vi "WS1050 BURN EFUSE Update.vi"() -> ()   [LabVIEW 2009]
panel:
  in  "A364X_VDD":refnum<visa-resource-name>="GPIB1::6::INSTR"
  in  "READBACK":bool
  out "error out 2":errorcluster
  out "Fuse Readback":string
  in  "BIT TO BURN":string="07450F"
  in  "stop":bool
  out "VISA resource name out":refnum<visa-resource-name>
  out "error out":errorcluster
  in  "error in (no error)":errorcluster
  in  "VISA resource name":refnum<visa-resource-name>="COM1"
  in  "PUSH BUTTON \nTO START TEST":bool
  # "TEST PROCEDURE TO BURN FUSE T7\n\n1. BIT TO BURN \"ENTER 0745XX\"\n2. INCREASE VDD TO 5V \"JUMPER THE YELLOW WIRE TO 5V\"\n3. DECREASE VDD TO 3.3V THEN MOVE JUMPER TO GND\n4. COMPLETED\n5. READ BACK TO VERIFY FUSE"
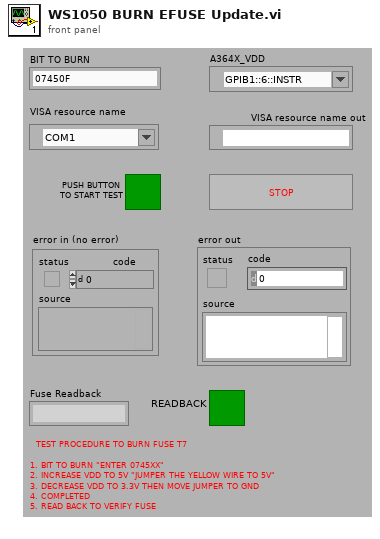
[diagram p1: front panel]
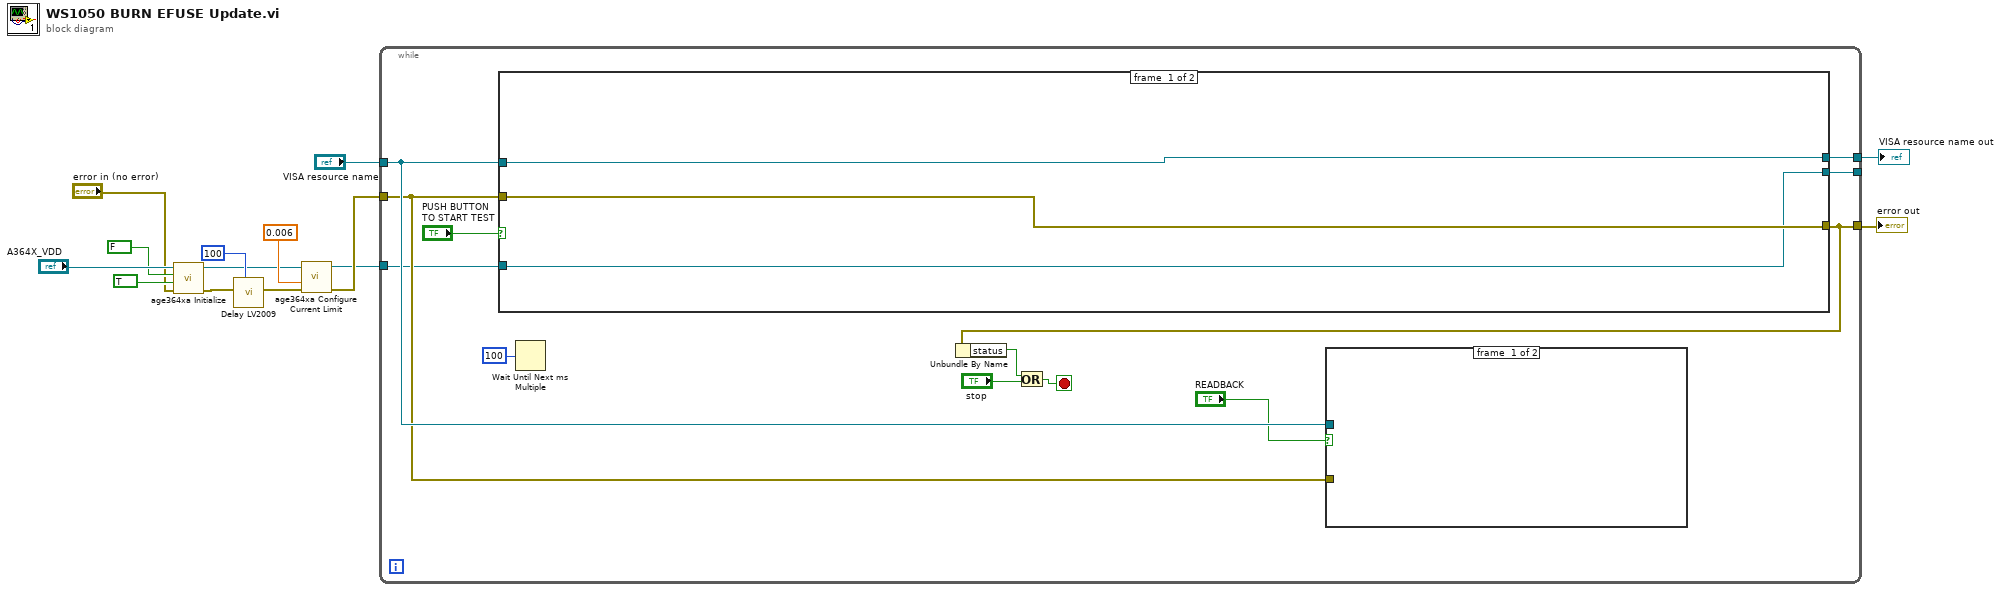
[diagram p0: block diagram]
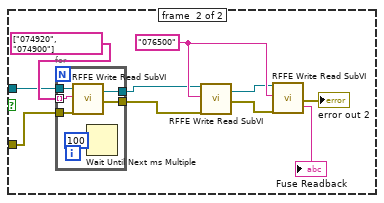
[diagram p2: hidden frame]
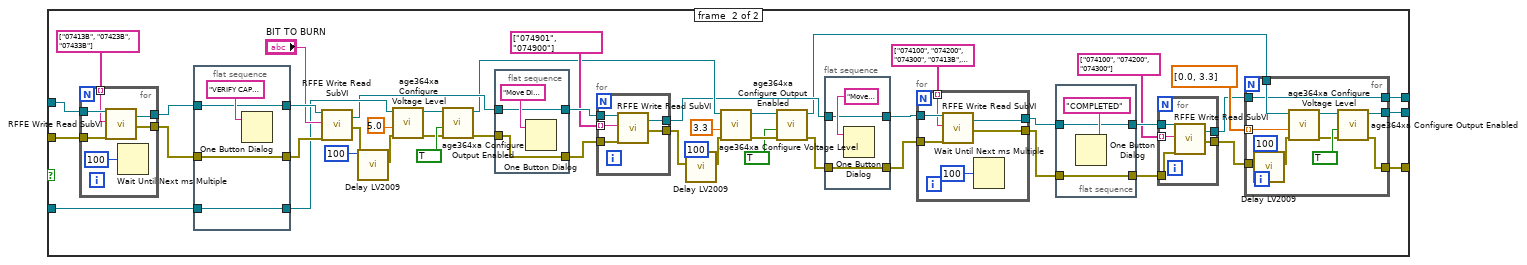
[diagram p3: hidden frame]
diagram:
  n1 = call "age364xa Initialize.vi"("error in (no error)"="error in (no error)", "ID Query (T: Query)"=TRUE, "Reset Device (T: Reset)"=FALSE, "Instrument Resource Name"="A364X_VDD") -> ("error out"=w8:errorcluster, "dup VISA session"=w7:refnum<visa-resource-name>)  [unwired: 6 in]
  n2 = call "Delay LV2009.vi"("milliseconds to wait"=u32 100, "error in (no error)"=w8) -> ("error out"=w10:errorcluster)  [unwired: 9 in]
  n3 = call "age364xa Configure Current Limit.vi"("error in (no error)"=w10, "Current Limit (0.0 Amps)"=0.006, "VISA session"=w7) -> ("error out"=w2:errorcluster, "dup VISA session"=w1:refnum<visa-resource-name>)  [unwired: 7 in]
  n4 = while {
    tunnel: "VISA resource name" -> [w19]
    tunnel: w2 -> [w18]
    tunnel: [w23] -> w12
    tunnel: [w25] -> w13
    tunnel: w1 -> [w16]
    tunnel: [w15] -> _
    stop <- w20 stop-if-true
    n5 = case shown="True" "PUSH BUTTON \nTO START TEST" {
      tunnel: w19 -> [w44 w92]
      tunnel: w18 -> [w45 w91]
      tunnel: [w45 w53] -> w23
      tunnel: [w44 w48] -> w25
      tunnel: w16 -> [w43 w74]
      tunnel: [w43 w47] -> w15
      frame #0 {
      }
      frame #1 {
        n6 = for {
          tunnel: w92 -> [w138]
          tunnel: w91 -> [w137]
          tunnel: string[] ["07413B", "07423B", "07433B"] -> [w136] mode=indexing
          tunnel: [w134] -> w89
          tunnel: [w133] -> w88
          n7 = call "RFFE Write Read SubVI.vi"("VISA resource name"=w138, "write buffer"=w136, "error in (no error)"=w137) -> ("VISA resource name out"=w133:refnum<visa-resource-name>, "error out"=w134:errorcluster)  [unwired: 12 in, 3 out]
          n8 = Wait Until Next ms Multiple(millisecond multiple=u32 100) -> ()  [unwired: 1 out]
        }
        n9 = flat-sequence {
          tunnel: w89 -> [w131]
          tunnel: [w131] -> w86
          tunnel: w88 -> [w130]
          tunnel: [w130] -> w87
          tunnel: [w129] -> w64
          tunnel: w74 -> [w129]
          frame #0 {
            n10 = One Button Dialog(message="VERIFY CAP ENTER BIT TO BURN") -> ()  [unwired: 1 in, 1 out]
          }
        }
        n11 = call "RFFE Write Read SubVI.vi"("VISA resource name"=w87, "write buffer"="BIT TO BURN", "error in (no error)"=w86) -> ("VISA resource name out"=w57:refnum<visa-resource-name>, "error out"=w67:errorcluster)  [unwired: 12 in, 3 out]
        n12 = call "Delay LV2009.vi"("milliseconds to wait"=u32 100, "error in (no error)"=w67) -> ("error out"=w69:errorcluster)  [unwired: 9 in]
        n13 = call "age364xa Configure Voltage Level.vi"("error in (no error)"=w69, "Level (0.0 Volts)"=5.0, "VISA session"=w64) -> ("error out"=w71:errorcluster, "dup VISA session"=w73:refnum<visa-resource-name>)  [unwired: 7 in]
        n14 = call "age364xa Configure Output Enabled.vi"("error in (no error)"=w71, "Output Enabled (F: Off)"=TRUE, "VISA session"=w73) -> ("error out"=w66:errorcluster, "dup VISA session"=w56:refnum<visa-resource-name>)  [unwired: 7 in]
        n15 = flat-sequence {
          tunnel: w57 -> [w127]
          tunnel: [w127] -> w84
          tunnel: w66 -> [w126]
          tunnel: [w126] -> w65
          frame #0 {
            n16 = One Button Dialog(message="Move Dig GND to +5V") -> ()  [unwired: 1 in, 1 out]
          }
        }
        n17 = for {
          tunnel: w84 -> [w125]
          tunnel: w65 -> [w124]
          tunnel: string[] ["074901", "074900"] -> [w123] mode=indexing
          tunnel: [w122] -> w54
          tunnel: [w121] -> w58
          n18 = call "RFFE Write Read SubVI.vi"("VISA resource name"=w125, "write buffer"=w123, "error in (no error)"=w124) -> ("VISA resource name out"=w122:refnum<visa-resource-name>, "error out"=w121:errorcluster)  [unwired: 12 in, 3 out]
        }
        n19 = call "Delay LV2009.vi"("milliseconds to wait"=u32 100, "error in (no error)"=w58) -> ("error out"=w63:errorcluster)  [unwired: 9 in]
        n20 = call "age364xa Configure Voltage Level.vi"("error in (no error)"=w63, "Level (0.0 Volts)"=3.3, "VISA session"=w56) -> ("error out"=w61:errorcluster, "dup VISA session"=w59:refnum<visa-resource-name>)  [unwired: 7 in]
        n21 = call "age364xa Configure Output Enabled.vi"("error in (no error)"=w61, "Output Enabled (F: Off)"=TRUE, "VISA session"=w59) -> ("error out"=w55:errorcluster, "dup VISA session"=w52:refnum<visa-resource-name>)  [unwired: 7 in]
        n22 = flat-sequence {
          tunnel: w55 -> [w119]
          tunnel: [w119] -> w75
          tunnel: w54 -> [w118]
          tunnel: [w118] -> w76
          frame #0 {
            n23 = One Button Dialog(message="Move JMP to GND") -> ()  [unwired: 1 in, 1 out]
          }
        }
        n24 = for {
          tunnel: w76 -> [w117]
          tunnel: w75 -> [w116]
          tunnel: string[] ["074100", "074200", "074300", "07413B", "07423B", "07433B"] -> [w115] mode=indexing
          tunnel: [w113] -> w80
          tunnel: [w112] -> w81
          n25 = call "RFFE Write Read SubVI.vi"("VISA resource name"=w117, "write buffer"=w115, "error in (no error)"=w116) -> ("VISA resource name out"=w112:refnum<visa-resource-name>, "error out"=w113:errorcluster)  [unwired: 12 in, 3 out]
          n26 = Wait Until Next ms Multiple(millisecond multiple=u32 100) -> ()  [unwired: 1 out]
        }
        n27 = flat-sequence {
          tunnel: w80 -> [w110]
          tunnel: [w110] -> w78
          tunnel: w81 -> [w109]
          tunnel: [w109] -> w79
          frame #0 {
            n28 = One Button Dialog(message="COMPLETED") -> ()  [unwired: 1 in, 1 out]
          }
        }
        n29 = for {
          tunnel: w79 -> [w108]
          tunnel: w78 -> [w107]
          tunnel: [w106] -> w50
          tunnel: [w105] -> w49
          tunnel: string[] ["074100", "074200", "074300"] -> [w104] mode=indexing
          n30 = call "RFFE Write Read SubVI.vi"("VISA resource name"=w108, "write buffer"=w104, "error in (no error)"=w107) -> ("VISA resource name out"=w105:refnum<visa-resource-name>, "error out"=w106:errorcluster)  [unwired: 12 in, 3 out]
        }
        n31 = for {
          tunnel: [w100] -> w47
          tunnel: [w99] -> w53
          tunnel: w52 -> [w98]
          tunnel: dbl[] [0.0, 3.3] -> [w96] mode=indexing
          tunnel: w50 -> [w95]
          tunnel: w49 -> [w93]
          tunnel: [w93] -> w48
          n32 = call "Delay LV2009.vi"("milliseconds to wait"=u32 100, "error in (no error)"=w95) -> ("error out"=w101:errorcluster)  [unwired: 9 in]
          n33 = call "age364xa Configure Voltage Level.vi"("error in (no error)"=w101, "Level (0.0 Volts)"=w96, "VISA session"=w98) -> ("error out"=w102:errorcluster, "dup VISA session"=w97:refnum<visa-resource-name>)  [unwired: 7 in]
          n34 = call "age364xa Configure Output Enabled.vi"("error in (no error)"=w102, "Output Enabled (F: Off)"=TRUE, "VISA session"=w97) -> ("error out"=w99:errorcluster, "dup VISA session"=w100:refnum<visa-resource-name>)  [unwired: 7 in]
        }
      }
    }
    n35 = Wait Until Next ms Multiple(millisecond multiple=u32 100) -> ()  [unwired: 1 out]
    n36 = Unbundle By Name(w23) -> ("status"=w22:bool)
    n37 = Or(x=w22, y="stop") -> (x .or. y?=w20:bool)
    n38 = case shown="True" "READBACK" {
      tunnel: w19 -> [_ w35]
      tunnel: w18 -> [_ w34]
      frame #0 {
      }
      frame #1 {
        w32 = "076500" ("write buffer")
        n39 = for {
          tunnel: w35 -> [w42]
          tunnel: w34 -> [w41]
          tunnel: string[] ["074920", "074900"] -> [w39] mode=indexing
          tunnel: [w38] -> w28
          tunnel: [w37] -> w29
          n40 = call "RFFE Write Read SubVI.vi"("VISA resource name"=w42, "write buffer"=w39, "error in (no error)"=w41) -> ("VISA resource name out"=w37:refnum<visa-resource-name>, "error out"=w38:errorcluster)  [unwired: 12 in, 3 out]
          n41 = Wait Until Next ms Multiple(millisecond multiple=u32 100) -> ()  [unwired: 1 out]
        }
        n42 = call "RFFE Write Read SubVI.vi"("VISA resource name"=w29, "write buffer"=w32, "error in (no error)"=w28) -> ("VISA resource name out"=w31:refnum<visa-resource-name>, "error out"=w30:errorcluster)  [unwired: 12 in, 3 out]
        n43 = call "RFFE Write Read SubVI.vi"("VISA resource name"=w31, "write buffer"=w32, "error in (no error)"=w30) -> ("Fuse Readback"=→"Fuse Readback":string, "error out"=→"error out 2":errorcluster)  [unwired: 12 in, 3 out]
      }
    }
  }
  "error out" <- w12
  "VISA resource name out" <- w13
